vi "subAcquisition_Info.vi"(3 "Stage Status":T1={" Current Position"=[-1.0, -12.0, 0.0], "Number of Axis"=3, "ILSID"=1}, 5 "Light control":T5={"Filter Set"=14, "Lasers DO"=[FALSE, FALSE, FALSE, FALSE, FALSE, FALSE, FALSE], "Lasers AO (V)"=[0.0, 0.0, 0.0, 0.0, 0.0, 0.0], "LED"=FALSE, "Global"=FALSE} {"Lasers AO (V)" min=0.0 max=5.0 step=0.01 scale=0.0..5.0 scale format="%#1.2f"; "Filter Set" items=["R-QuasAr", "R-Cy5", "R-mCherry", "R-mOrange", "R-GFP", "R-CFP/DAPI", "R-BFP", "R-LED", "SDC-Cy5", "SDC-mCherry", "SDC-mO2", "SDC-GFP", "SDC-CFP/DAPI", "SDC-BFP", "SDC-LED"]}, 7 "Image Info":T2={"Status"="Ready", "scale bar (μm)"=inf, "Image"=array1024x1024[1048576 elements], "Histogram"={"max value"=453, "mean"=398, "min value"=349, "Histogram"={"X Values"=[349.52, 350.56, 351.6, 352.64000000000004, 353.68000000000006, 354.7200000000001, 355.7600000000001, 356.8000000000001, 357.84000000000015, 358.88000000000017, 359.9200000000002, 360.9600000000002, 362.0000000000002, 363.04000000000025, 364.08000000000027, 365.1200000000003, 366.1600000000003, 367.20000000000033, 368.24000000000035, 369.28000000000037, 370.3200000000004, 371.3600000000004, 372.40000000000043, 373.44000000000045, 374.4800000000005, 375.5200000000005, 376.5600000000005, 377.60000000000053, 378.64000000000055, 379.6800000000006, 380.7200000000006, 381.7600000000006, 382.80000000000064, 383.84000000000066, 384.8800000000007, 385.9200000000007, 386.9600000000007, 388.00000000000074, 389.04000000000076, 390.0800000000008, 391.1200000000008, 392.1600000000008, 393.20000000000084, 394.24000000000086, 395.2800000000009, 396.3200000000009, 397.3600000000009, 398.40000000000094, 399.44000000000096, 400.480000000001, 401.520000000001, 402.560000000001, 403.60000000000105, 404.64000000000107, 405.6800000000011, 406.7200000000011, 407.7600000000011, 408.80000000000115, 409.84000000000117, 410.8800000000012, 411.9200000000012, 412.96000000000123, 414.00000000000125, 415.04000000000127, 416.0800000000013, 417.1200000000013, 418.16000000000133, 419.20000000000135, 420.2400000000014, 421.2800000000014, 422.3200000000014, 423.36000000000143, 424.40000000000146, 425.4400000000015, 426.4800000000015, 427.5200000000015, 428.56000000000154, 429.60000000000156, 430.6400000000016, 431.6800000000016, 432.7200000000016, 433.76000000000164, 434.80000000000166, 435.8400000000017, 436.8800000000017, 437.9200000000017, 438.96000000000174, 440.00000000000176, 441.0400000000018, 442.0800000000018, 443.1200000000018, 444.16000000000184, 445.20000000000186, 446.2400000000019, 447.2800000000019, 448.3200000000019, 449.36000000000195, 450.40000000000197, 451.440000000002, 452.480000000002], "Histogram: h(x)"=[1, 0, 1, 0, 0, 0, 0, 1, 0, 2, 3, 0, 0, 0, 1, 1, 0, 4, 9, 8, 10, 21, 26, 28, 34, 154, 119, 176, 194, 271, 421, 601, 667, 990, 1403, 1876, 2665, 3703, 4776, 6660, 8548, 10841, 13082, 15767, 17625, 19251, 20235, 20235, 19157, 17812, 28764, 10625, 8397, 6381, 4845, 3578, 2694, 2049, 1523, 1242, 990, 763, 618, 513, 389, 301, 229, 180, 164, 124, 79, 59, 40, 39, 27, 44, 17, 16, 13, 9, 8, 6, 5, 7, 5, 2, 1, 1, 2, 1, 2, 5, 2, 1, 0, 0, 0, 3, 0, 2]}}, "Scale Info"={"Pixel size (nm)"=inf, "Total x width (μm)"=inf, "Total y width (μm)"=inf}, "Camera View indicator"=array1024x1024[1048576 elements], "max frame rate (Hz)"=200.0}, 8 "Confocal scanner":T7={"SDC shutter"=FALSE, "FWPosition"=3, "FW speed"=3, "Disk spinning?"=FALSE, "Disk speed (rpm)"=4000.0} {"Disk speed (rpm)" min=1500.0 max=10000.0; "FW speed" min=1 max=3 step=1; "FWPosition" items=["CFP"=1, "GFP"=2, "mCherry"=3, "Alexa647"=4, "OFP"=5, "- empty 6 -"=6]}, 9 "TI-Ctrl":T6={"Obj"=6, "Cube Bottom"=1, "Cube Top"=4, "PFS-Ctrl"={"PFS IO"=FALSE, "PSF Err"=FALSE, "PSF Pos"=0}, "Z-Ctrl"={"Z-pos"=499.75, "Home"=TRUE, "Sensitivity"=1}, "Condenser"=2, "Lightpath"=enum."EYE"} {"Condenser" items=["A"=1, "DICN2"=2, "- empty 3 -"=3, "- empty 4 -"=4, "- empty 5 -"=5, "- empty 6 -"=6]; "Z-Ctrl"."Sensitivity" min=1 max=3 step=1 scale=1.0..3.0; "PFS-Ctrl"."PSF Pos" scale=0.0..16400.0; "Cube Top" items=["Cy5"=1, "TxRed"=2, "mO2"=3, "GFP-B"=4, "DAPI"=5, "- empty 6 -"=6]; "Cube Bottom" items=["- empty 1 -"=1, "- empty 2 -"=2, "- empty 3 -"=3, "- empty 4 -"=4, "- empty 5 -"=5, "- empty 6 -"=6]; "Obj" items=["20x/.75 Dry PFS"=1, " 40x/1.3 Oil PFS"=2, "60x/1.4 Oil PFS"=3, "- empty 4 -"=4, "- empty 5 -"=5, "- empty 6 -"=6]}, 10 "Camera Info":T3={"Camera Details Array"=[{"Model"="C11440-22C", "Camera ID"="S/N: 003223", "Firmware"="3.20.A"}], "Handle"=0, "Camera in use "={"Model"="C11440-22C", "Camera ID"="S/N: 003223", "Bits"=16}}, 11 "Camera Ctrl":T4={"Chosen Camera"=0, "ROI selection"=0, "Live"=FALSE, "ROI define"=FALSE, "Snap"=FALSE, "ROI update"=FALSE, "ROI previous "=FALSE, "ROI"={"Bin"=2, "ROI"={"x offset"=256, "y offset"=256, "x width"=512, "y width"=512}}, "Exposure (ms)"=100.0, "Symmetrical"=FALSE, "Autoscale"=FALSE, "Scale"={"Scale.Min"=0, "Scale.Max"=6038}} {"Scale"."Scale.Max" min=1 max=5000 step=1; "Scale"."Scale.Min" min=1 max=5000 step=1; "Exposure (ms)" min=1.0 max=5000.0 step=1.0; "ROI"."ROI"."x offset" min=1 max=512 step=1; "ROI"."ROI"."y offset" min=1 max=512 step=1; "ROI"."ROI"."x width" min=1 max=512 step=1; "ROI"."ROI"."y width" min=1 max=512 step=1; "ROI"."Bin" items=["1x1"=1, "2x2"=2, "4x4"=4]; "ROI selection" items=["Full ROI", "Central quad", "Confocal"]; "Chosen Camera" items=["Left", "Right"]}) -> (2 "Text":string="nrow = \t240\rncol = \t192\rrow offset = \t896\rcol offset = \t784\rBinning =\t1\r============== \r594nm eff. =\t1.000000\r Exposure (msec) =\t0\r------------- \r488 weak eff. =\t0.000000\r Exposure (msec) =\t1\r------------- \rEmission filter =\tET575/50\r============== ")   [LabVIEW 2015]
panel:
  # "X"
  # "Y"
  # "Red"
  # "637"
  # "561"
  # "488"
  # "405"
  # "532"
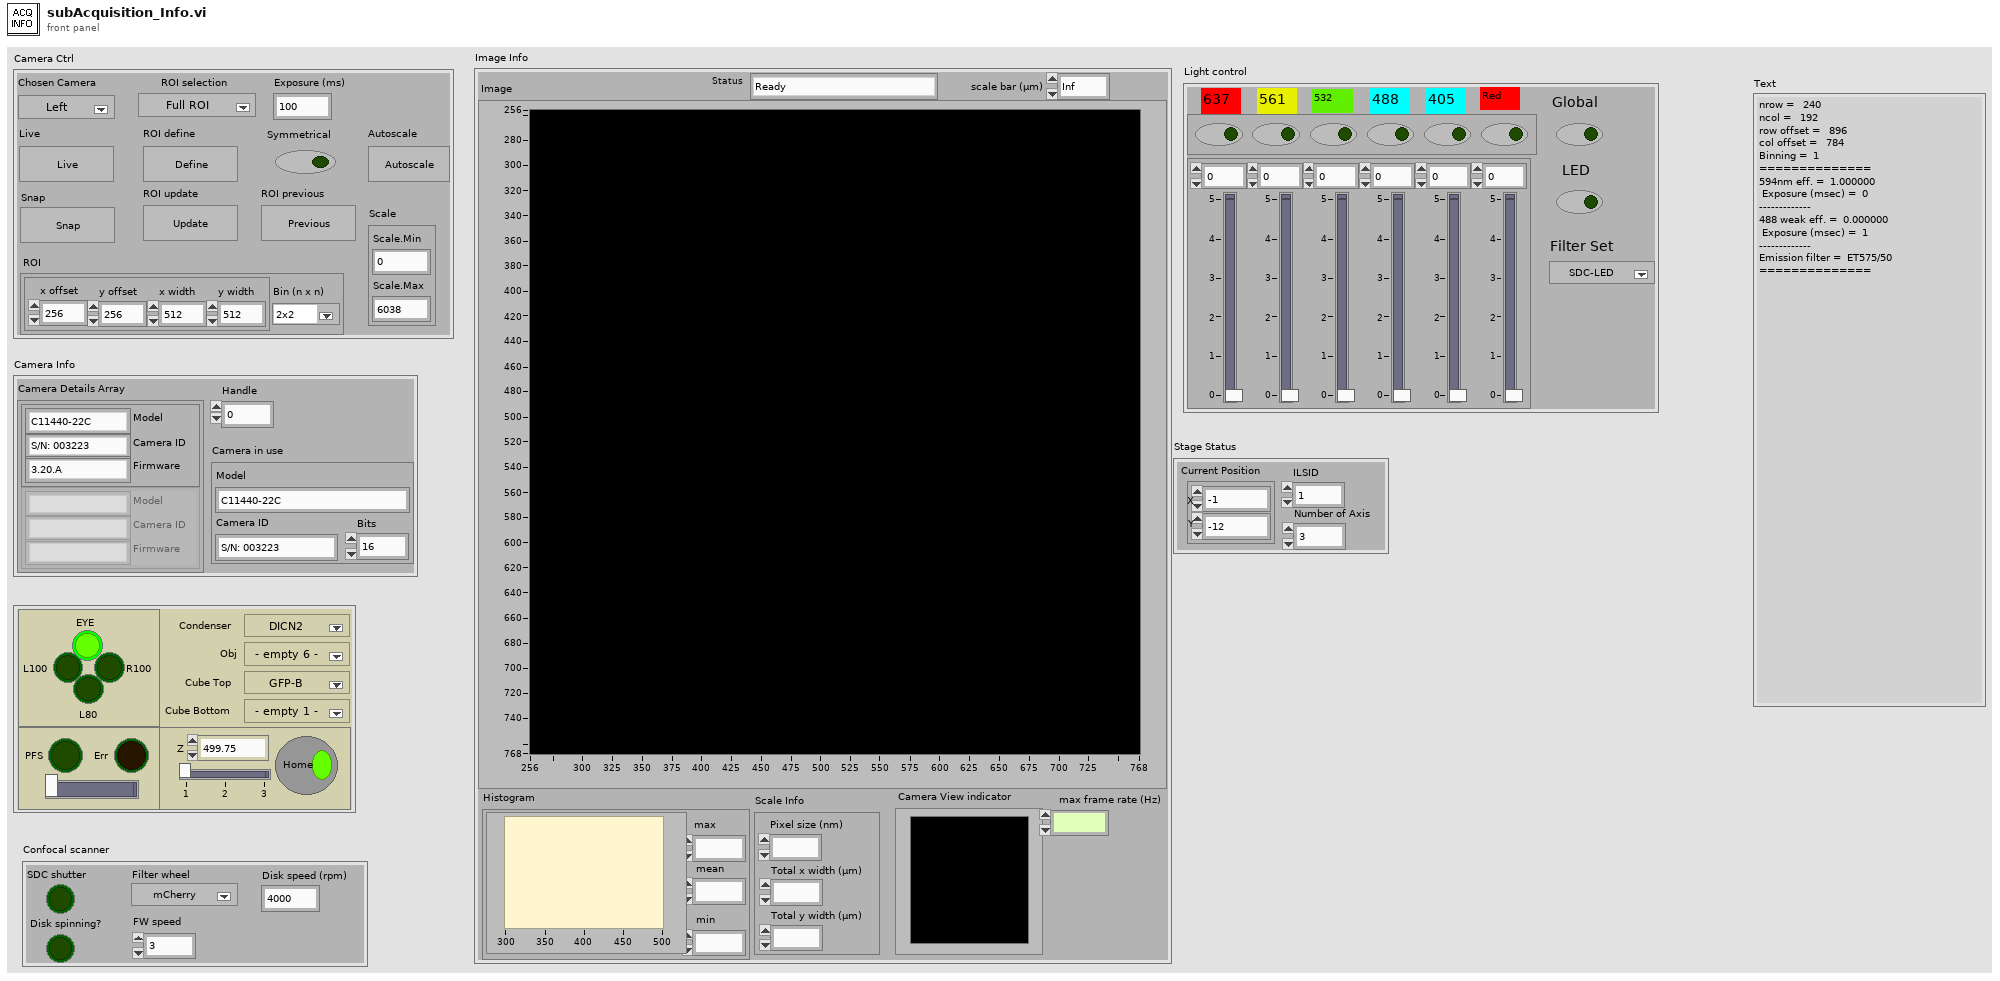
[diagram p1: front panel]
types:
  T1 = cluster{" Current Position":dbl[], "Number of Axis":i32, "ILSID":i32}
  T2 = cluster{"Status":string, "scale bar (μm)":dbl, "Image":u16[][], "Histogram":cluster{"max value":u16, "mean":i16, "min value":u16, "Histogram":cluster{"X Values":dbl[], "Histogram: h(x)":i32[]}}, "Scale Info":cluster{"Pixel size (nm)":dbl, "Total x width (μm)":dbl, "Total y width (μm)":dbl}, "Camera View indicator":u16[][], "max frame rate (Hz)":dbl}
  T3 = cluster{"Camera Details Array":cluster{"Model":string, "Camera ID":string, "Firmware":string}[], "Handle":u32, "Camera in use ":cluster{"Model":string, "Camera ID":string, "Bits":i32}}
  T4 = cluster{"Chosen Camera":u32, "ROI selection":u16, "Live":bool, "ROI define":bool, "Snap":bool, "ROI update":bool, "ROI previous ":bool, "ROI":cluster{"Bin":u16, "ROI":cluster{"x offset":i32, "y offset":i32, "x width":i32, "y width":i32}}, "Exposure (ms)":dbl, "Symmetrical":bool, "Autoscale":bool, "Scale":cluster{"Scale.Min":i32, "Scale.Max":i32}}
  T5 = cluster{"Filter Set":i32, "Lasers DO":bool[], "Lasers AO (V)":dbl[], "LED":bool, "Global":bool}
  T6 = cluster{"Obj":u16, "Cube Bottom":u16, "Cube Top":u16, "PFS-Ctrl":cluster{"PFS IO":bool, "PSF Err":bool, "PSF Pos":u32}, "Z-Ctrl":cluster{"Z-pos":dbl, "Home":bool, "Sensitivity":u8}, "Condenser":u16, "Lightpath":enum32{"EYE", "L100", "R100", "L80"}}
  T7 = cluster{"SDC shutter":bool, "FWPosition":i32, "FW speed":i32, "Disk spinning?":bool, "Disk speed (rpm)":dbl}
  T8 = cluster{"Model":string, "Camera ID":string, "Bits":i32}
  T9 = cluster{"Pixel size (nm)":dbl, "Total x width (μm)":dbl, "Total y width (μm)":dbl}
  T10 = cluster{"Bin":u16, "ROI":cluster{"x offset":i32, "y offset":i32, "x width":i32, "y width":i32}}
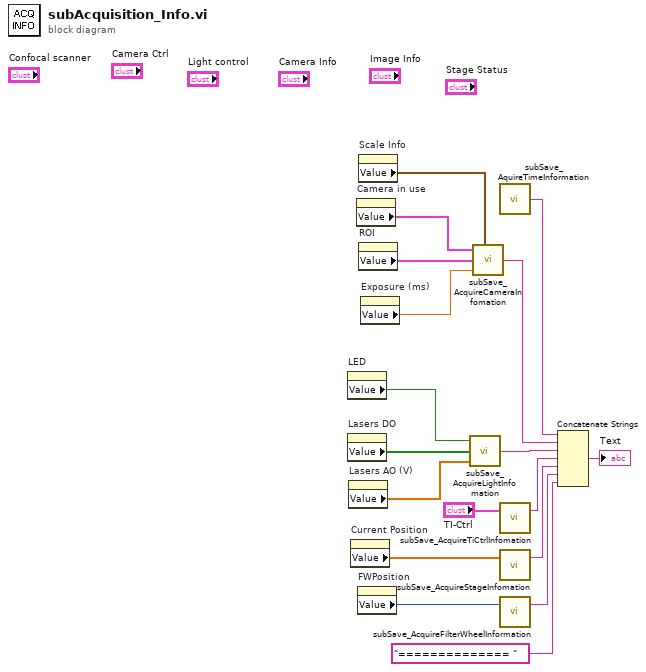
[diagram p0: block diagram]
diagram:
  n1 = property on="LED" class="Bool (strict)"() -> ("Value"=w7:bool)  [unwired: 2 in, 2 out]
  n2 = property on="Lasers DO" class="Arr (strict)"() -> ("Value"=w6:bool[])  [unwired: 2 in, 2 out]
  n3 = property on="Lasers AO (V)" class="Arr (strict)"() -> ("Value"=w5:dbl[])  [unwired: 2 in, 2 out]
  n4 = property on="Current Position" class="Arr (strict)"() -> ("Value"=w4:dbl[])  [unwired: 2 in, 2 out]
  n5 = property on="Camera in use" class="Clust (strict)"() -> ("Value"=w2:T8)  [unwired: 2 in, 2 out]
  n6 = property on="FWPosition" class="Ring (strict)"() -> ("Value"=w3:i32)  [unwired: 2 in, 2 out]
  n7 = property on="Scale Info" class="Clust (strict)"() -> ("Value"=w8:T9)  [unwired: 2 in, 2 out]
  n8 = property on="ROI" class="Clust (strict)"() -> ("Value"=w9:T10)  [unwired: 2 in, 2 out]
  n9 = property on="Exposure (ms)" class="DigNum (strict)"() -> ("Value"=w1:dbl)  [unwired: 2 in, 2 out]
  n10 = call "subSave_AcquireLightInfomation.vi"("AO (V)"=w5, "DO"=w6, "LED"=w7) -> ("Text out"=w11:string)
  n11 = call "subSave_AcquireCameraInfomation.vi"("Camera in use"=w2, "Scale Info"=w8, "ROI"=w9, "Exposure (msec)"=w1) -> ("Text Out"=w10:string)  [unwired: 1 in]
  n12 = call "subSave_AquireTimeInformation.vi"() -> ("time out"=w17:string)  [unwired: 1 in]
  n13 = call "subSave_AcquireTiCtrlInfomation.vi"("TI-Ctrl"="TI-Ctrl") -> ("Text out"=w15:string)  [unwired: 2 in]
  n14 = call "subSave_AcquireStageInfomation.vi"("Positions"=w4) -> ("Text out"=w14:string)  [unwired: 2 in]
  n15 = call "subSave_AcquireFilterWheelInformation.vi"("FWPosition"=w3) -> ("FW text"=w13:string)  [unwired: 2 in]
  n16 = Concatenate Strings(w17, w10, w11, w15, w14, w13, "============== " ("string")) -> (→"Text":string)
